vi "csm_lumikki_instron_initRamp_poller.vi"   [LabVIEW 2009]
types:
  T1 = cluster{"Name":string, "Type":i32, "SI Full Scale":dbl, "Full Scale":dbl, "Units String":string, "Display Format":string, "Gauge Length":dbl}[][]
  T2 = cluster{"Device ID":i32, "Device Name":string, "Device Type":i32}[]
  T3 = cluster{"Set Point Time":dbl, "Set Point Time":dbl, "Double":dbl, "Double":dbl}
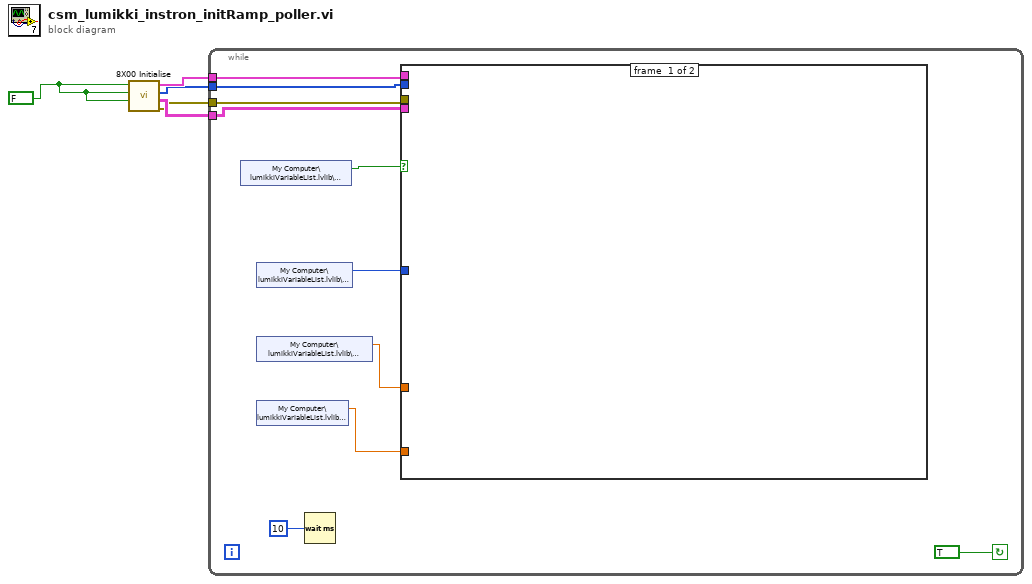
[diagram p0: block diagram]
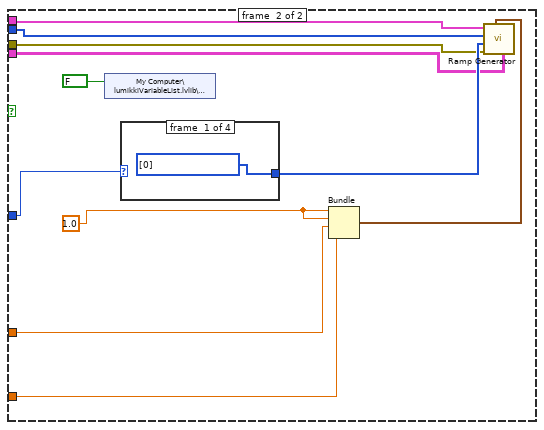
[diagram p2: hidden frame]
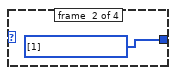
[diagram p3: hidden frame]
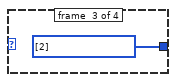
[diagram p4: hidden frame]
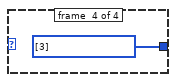
[diagram p5: hidden frame]
diagram:
  w1 = FALSE ("Reset?")
  n1 = call "8X00 Initialise.vi"("Reset?"=w1, "Create DVM? (T)"=w1, "Create Console? (T)"=w1) -> ("error out"=w2:errorcluster, "Channel Data"=w5:T1, "Axis Selector"=w3:i32[], "Axis Information"=w4:T2)  [unwired: 1 in]
  n2 = while {
    tunnel: w5 -> [w12]
    tunnel: w4 -> [w13]
    tunnel: w3 -> [w14]
    tunnel: w2 -> [w11]
    stop <- TRUE continue-if-true
    n3 = shared-variable "My Computer\\lumikkiVariableList.lvlib\\startSetRamp"() -> (w10:bool)  [unwired: 1 in, 1 out]
    n4 = shared-variable "My Computer\\lumikkiVariableList.lvlib\\channelInt"() -> (w7:i32)  [unwired: 1 in, 1 out]
    n5 = shared-variable "My Computer\\lumikkiVariableList.lvlib\\rampAmplitude"() -> (w9:dbl)  [unwired: 1 in, 1 out]
    n6 = shared-variable "My Computer\\lumikkiVariableList.lvlib\\rampRate"() -> (w8:dbl)  [unwired: 1 in, 1 out]
    n7 = Wait (ms)(milliseconds to wait=u32 10) -> ()  [unwired: 1 out]
    n8 = case shown="True" w10 {
      tunnel: w14 -> [_ w23]
      tunnel: w13 -> [_ w22]
      tunnel: w12 -> [_ w21]
      tunnel: w11 -> [_ w20]
      tunnel: w9 -> [_ w19]
      tunnel: w8 -> [_ w18]
      tunnel: w7 -> [_ w17]
      frame #0 {
      }
      frame #1 {
        w26 = 1.0 ("Set Point Time")
        n9 = shared-variable "My Computer\\lumikkiVariableList.lvlib\\startSetRamp"(FALSE ("startSetRamp")) -> ()  [unwired: 1 in, 1 out]
        n10 = case shown="1, Default" w17 {
          tunnel: [w27 w28 w29 w30] -> w25
          frame #0 {
            w27 = u16[] [0] items=["Channel 1", "Channel 2", "Channel 3", "Channel 4"] ("Choose channel to apply\nthe setpoint")
          }
          frame #1 {
            w28 = u16[] [1] items=["Channel 1", "Channel 2", "Channel 3", "Channel 4"] ("Choose channel to apply\nthe setpoint")
          }
          frame #2 {
            w29 = u16[] [2] items=["Channel 1", "Channel 2", "Channel 3", "Channel 4"] ("Choose channel to apply\nthe setpoint")
          }
          frame #3 {
            w30 = u16[] [3] items=["Channel 1", "Channel 2", "Channel 3", "Channel 4"] ("Choose channel to apply\nthe setpoint")
          }
        }
        n11 = Bundle("Set Point Time"=w26, "Set Point Time"=w26, "Double"=w19, "Double"=w18) -> (w24:T3)  [unwired: 1 in]
        n12 = call "Ramp Generator.vi"("Channel Data"=w21, "Input cluster"=w24, "error in (no error)"=w20, "Channels"=w25, "Axis Selector"=w23, "Axis Information"=w22) -> ()  [unwired: 2 in, 4 out]
      }
    }
  }
